vi "List Rules as Strings.vi"(8 "error in (no error)":errorcluster, 11 "GlobalLogFilter In":refnum<class "LogFilter.lvclass">) -> (0 "error out":errorcluster, 2 "Rule Strings":string[](array[string]), 3 "GlobalLogFilter Out":refnum<class "LogFilter.lvclass">)   [LabVIEW 2017, in "CSM File Logger.lvlib"]
doc: "### List Rules as Strings.vi\n\n-- <b>Controls</b> --\n- <b>GlobalLogFilter in</b>:\n\n-- <b>Indicators</b> --\n- <b>Rule Strings</b>:\n- <b>GlobalLogFilter out</b>:"
uses:
  CSM File Logger.lvlib
  _Support/GlobalEvent/LogFilter/LogFilter.lvclass
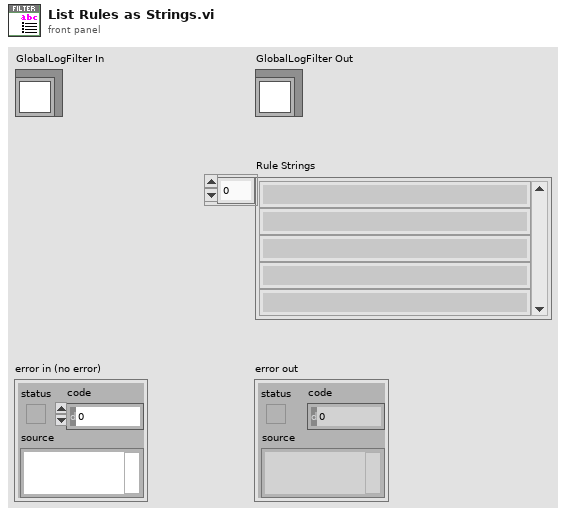
[diagram p1: front panel]
types:
  T1 = typedef "Communicable State Machine.lvlib/_CSM_GlobalLog Filter Rules - v1.2.ctl" = cluster{"Global":cluster{"CSM":string[], "LogType":T2[], "State":string[], "StateType":T3[], "Broadcast":string[], "UserLog":string[]}, "CSM":cluster{"LogType":cluster{"CSM":string, "LogType":T2}[], "State":cluster{"CSM":string, "State":string}[], "StateType":cluster{"CSM":string, "LogType":T3}[], "Broadcast":cluster{"CSM":string, "Broadcast":string}[], "UserLog":cluster{"CSM":string, "UserLog":string}[]}, "PeriodicMessageFilter":cluster{"Enable":bool, "Threshold(#/s)":dbl, "CheckPeriod(s)":dbl}}
  T2 = typedef "Communicable State Machine.lvlib/_CSM_GlobalLog_MSG_TYPE.ctl" = enum16{"User Log", "State Change", "Status", "Interrupt", "Register", "Unregister", "Error Log", "Module Created", "Module Destroyed", "Async Message", "No-Rep Async Message", "Sync Message", "AsyncMsg Complete", "SyncMsg Complete"}
  T3 = typedef "Communicable State Machine.lvlib/_CSM_GlobalLog_STATE_TYPE.ctl" = enum16{"State - Internal State", "State - External Message", "State - Response", "State - Complete"}
  T4 = cluster{"Enable":bool, "Threshold(#/s)":dbl, "CheckPeriod(s)":dbl}
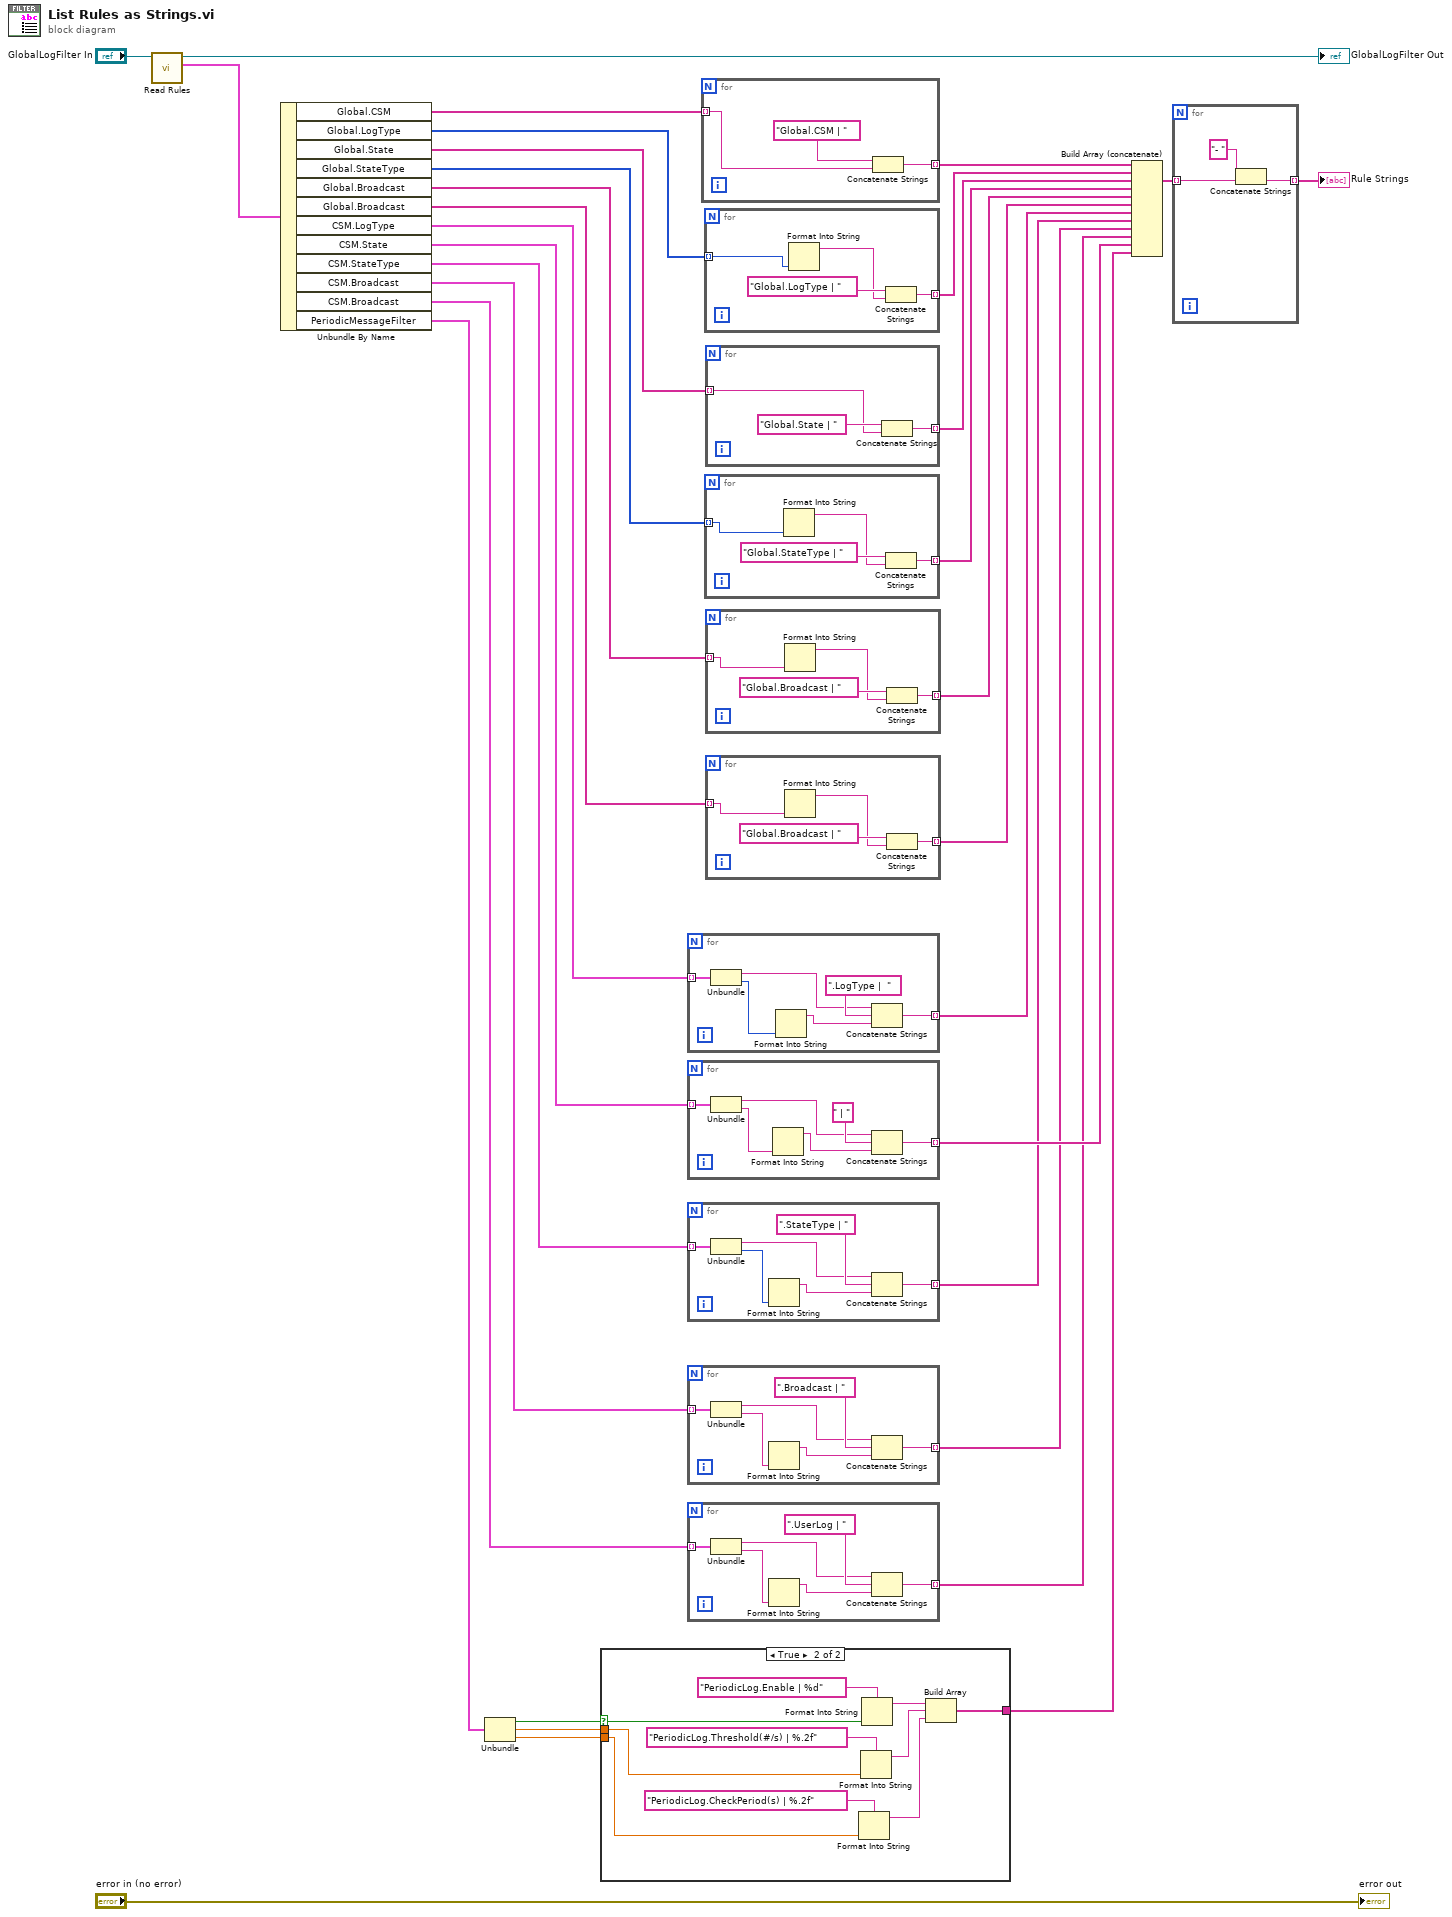
[diagram p0: block diagram]
diagram:
  n1 = call "Read Rules.vi"("LogFilter In"="GlobalLogFilter In") -> ("Rules"=w14:T1, "LogFilter Out"=→"GlobalLogFilter Out":refnum<class "LogFilter.lvclass">)  [unwired: 8 in, 1 out]
  n2 = Unbundle By Name(w14) -> ("Global.CSM"=w31:string[], "Global.LogType"=w29:T2[], "Global.State"=w27:string[], "Global.StateType"=w19:T3[], "Global.Broadcast"=w8:string[], "Global.Broadcast"=w4:string[], "CSM.LogType"=w25:cluster{"CSM":string, "LogType":T2}[], "CSM.State"=w23:cluster{"CSM":string, "State":string}[], "CSM.StateType"=w17:cluster{"CSM":string, "LogType":T3}[], "CSM.Broadcast"=w6:cluster{"CSM":string, "Broadcast":string}[], "CSM.Broadcast"=w2:cluster{"CSM":string, "Broadcast":string}[], "PeriodicMessageFilter"=w13:T4)
  n3 = Unbundle(w13) -> ("Enable"=w12:bool, "Threshold(#/s)"=w11:dbl, "CheckPeriod(s)"=w10:dbl)
  n4 = case shown="True" w12 {
    selector: w12 -> [_ w43]
    tunnel: w11 -> [_ w40]
    tunnel: w10 -> [_ w38]
    tunnel: [_ w34] -> w9
    frame False {
    }
    frame True {
      n5 = Format Into String(format string="PeriodicLog.CheckPeriod(s) | %.2f", w38) -> (resulting string=w35:string)  [unwired: 2 in, 1 out]
      n6 = Format Into String(format string="PeriodicLog.Threshold(#/s) | %.2f", w40) -> (resulting string=w36:string)  [unwired: 2 in, 1 out]
      n7 = Format Into String(format string="PeriodicLog.Enable | %d", w43) -> (resulting string=w37:string)  [unwired: 2 in, 1 out]
      n8 = Build Array(w37, w36, w35) -> (w34:string[])
    }
  }
  n9 = for {
    tunnel: w25 -> [w47] mode=indexing
    tunnel: [w48] -> w24 mode=indexing
    n10 = Unbundle(w47) -> ("CSM"=w46:string, "LogType"=w45:T2)
    n11 = Format Into String(w45) -> (resulting string=w44:string)  [unwired: 3 in, 1 out]
    n12 = Concatenate Strings(w46, ".LogType |  " ("string"), w44) -> (w48:string)
  }
  n13 = for {
    tunnel: w23 -> [w53] mode=indexing
    tunnel: [w54] -> w22 mode=indexing
    n14 = Unbundle(w53) -> ("CSM"=w52:string, "State"=w51:string)
    n15 = Format Into String(w51) -> (resulting string=w50:string)  [unwired: 3 in, 1 out]
    n16 = Concatenate Strings(w52, " | " ("string"), w50) -> (w54:string)
  }
  n17 = for {
    tunnel: w17 -> [w59] mode=indexing
    tunnel: [w60] -> w16 mode=indexing
    n18 = Unbundle(w59) -> ("CSM"=w58:string, "LogType"=w57:T3)
    n19 = Format Into String(w57) -> (resulting string=w56:string)  [unwired: 3 in, 1 out]
    n20 = Concatenate Strings(w58, ".StateType | " ("string"), w56) -> (w60:string)
  }
  n21 = for {
    tunnel: w6 -> [w65] mode=indexing
    tunnel: [w66] -> w5 mode=indexing
    n22 = Unbundle(w65) -> ("CSM"=w64:string, "Broadcast"=w63:string)
    n23 = Format Into String(w63) -> (resulting string=w62:string)  [unwired: 3 in, 1 out]
    n24 = Concatenate Strings(w64, ".Broadcast | " ("string"), w62) -> (w66:string)
  }
  n25 = for {
    tunnel: w2 -> [w71] mode=indexing
    tunnel: [w72] -> w1 mode=indexing
    n26 = Unbundle(w71) -> ("CSM"=w70:string, "Broadcast"=w69:string)
    n27 = Format Into String(w69) -> (resulting string=w68:string)  [unwired: 3 in, 1 out]
    n28 = Concatenate Strings(w70, ".UserLog | " ("string"), w68) -> (w72:string)
  }
  n29 = for {
    tunnel: w31 -> [w75] mode=indexing
    tunnel: [w74] -> w30 mode=indexing
    n30 = Concatenate Strings("Global.CSM | " ("string"), w75) -> (w74:string)
  }
  n31 = for {
    tunnel: w29 -> [w78] mode=indexing
    tunnel: [w79] -> w28 mode=indexing
    n32 = Format Into String(w78) -> (resulting string=w77:string)  [unwired: 3 in, 1 out]
    n33 = Concatenate Strings("Global.LogType | " ("string"), w77) -> (w79:string)
  }
  n34 = for {
    tunnel: w19 -> [w82] mode=indexing
    tunnel: [w83] -> w18 mode=indexing
    n35 = Format Into String(w82) -> (resulting string=w81:string)  [unwired: 3 in, 1 out]
    n36 = Concatenate Strings("Global.StateType | " ("string"), w81) -> (w83:string)
  }
  n37 = for {
    tunnel: w27 -> [w85] mode=indexing
    tunnel: [w86] -> w26 mode=indexing
    n38 = Concatenate Strings("Global.State | " ("string"), w85) -> (w86:string)
  }
  n39 = for {
    tunnel: w8 -> [w89] mode=indexing
    tunnel: [w90] -> w7 mode=indexing
    n40 = Format Into String(w89) -> (resulting string=w88:string)  [unwired: 3 in, 1 out]
    n41 = Concatenate Strings("Global.Broadcast | " ("string"), w88) -> (w90:string)
  }
  n42 = for {
    tunnel: w4 -> [w93] mode=indexing
    tunnel: [w94] -> w3 mode=indexing
    n43 = Format Into String(w93) -> (resulting string=w92:string)  [unwired: 3 in, 1 out]
    n44 = Concatenate Strings("Global.Broadcast | " ("string"), w92) -> (w94:string)
  }
  n45 = Build Array (concatenate)(w30, w28, w26, w18, w7, w3, w24, w16, w5, w1, w22, w9) -> (w20:string[])
  n46 = for {
    tunnel: [w96] -> w21 mode=indexing
    tunnel: w20 -> [w97] mode=indexing
    n47 = Concatenate Strings("- " ("string"), w97) -> (w96:string)
  }
  "Rule Strings" <- w21
  "error out" <- "error in (no error)"
